vi "Initialize Step Result.vi"(8 "error in (no error)":errorcluster) -> (0 "error out":errorcluster, 3 "New Step Result":T1, 4 "current time":timestamp)   [LabVIEW 2015]
uses:
  Controls/Step Result.ctl
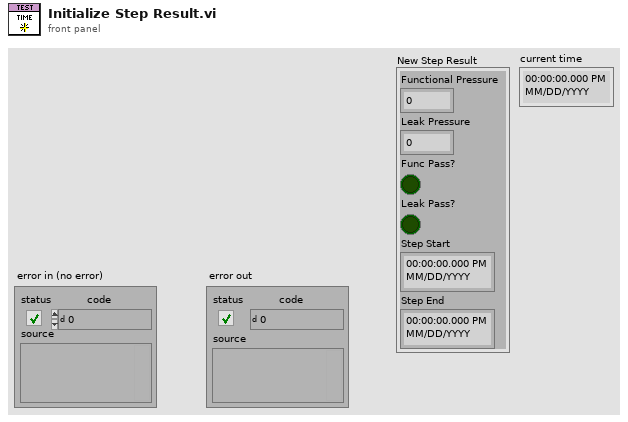
[diagram p1: front panel]
types:
  T1 = typedef "Step Result.ctl" = cluster{"Functional Pressure":dbl, "Leak Pressure":dbl, "Func Pass?":bool, "Leak Pass?":bool, "Step Start":timestamp, "Step End":timestamp}
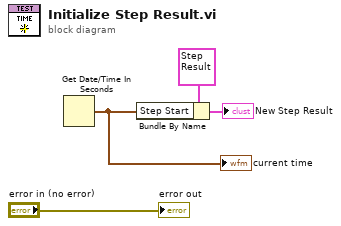
[diagram p0: block diagram]
diagram:
  n1 = Get Date/Time In Seconds() -> (seconds since 1Jan1904=w3:timestamp)
  "current time" <- w3
  n2 = Bundle By Name(cluster=T1 {"Functional Pressure"=0.0, "Leak Pressure"=0.0, "Func Pass?"=FALSE, "Leak Pass?"=FALSE, "Step Start"=timestamp(0 s since 1904-01-01), "Step End"=timestamp(0 s since 1904-01-01)} ("Step Result"), "Step Start"=w3) -> (→"New Step Result":T1)
  "error out" <- "error in (no error)"
